vi "newfinal.vi"(8 "error in (no error)":errorcluster, 11 "output cluster in":T1) -> (0 "error out":errorcluster, 3 "output cluster out":T1)   [LabVIEW 2013]
uses:
  calib_Sub_Typdef.ctl
  ScreenCam2_TypDEf.ctl
  CamAndObj_TypDEf.ctl
  ROIInfo_TypDef.ctl
  calibPixel.ctl
  2DTypDef.ctl
  CamRoiTypDef.ctl
  finalCalibTypdef.ctl
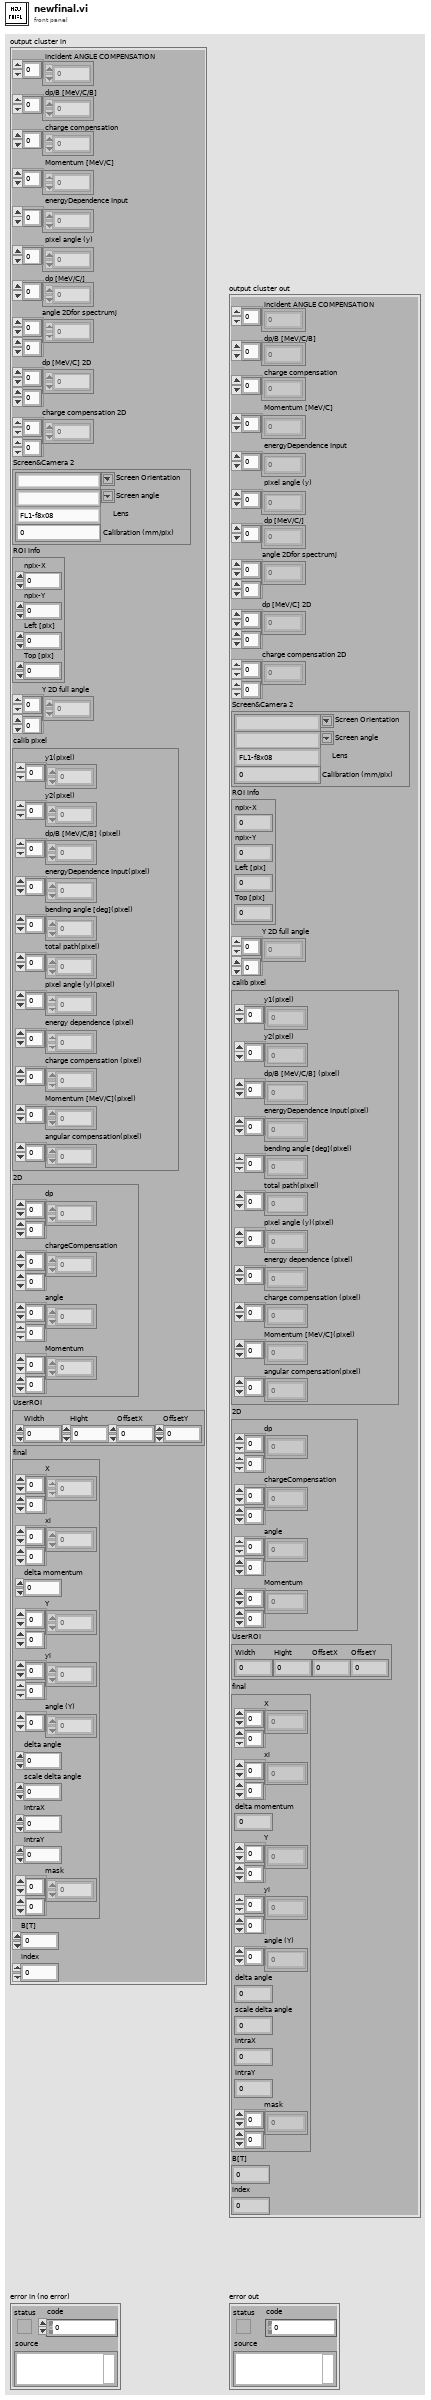
[diagram p1: front panel]
types:
  T1 = typedef "calib_Sub_Typdef.ctl" = cluster{"incident ANGLE COMPENSATION":dbl[], "dp/B [MeV/C/B]":dbl[], "charge compensation":dbl[], "Momentum [MeV/C]":dbl[], "energyDependence Input":dbl[], "pixel angle (y)":dbl[], "dp [MeV/C/] ":dbl[], "angle 2Dfor spectrumj":dbl[][], "dp [MeV/C] 2D":dbl[][], "charge compensation 2D":dbl[][], "Screen&Camera 2":T2, "ROI info":T4, "Y 2D full angle":dbl[][], "calib pixel":T5, "2D":T6, "UserROI":T7, "final":T8, "B[T]":dbl, "index":dbl}
  T2 = typedef "ScreenCam2_TypDEf.ctl" = cluster{"Screen Orientation":string, "Screen angle":string, "Lens":T3, "Calibration (mm/pix)":dbl}
  T3 = typedef "CamAndObj_TypDEf.ctl" = enum16{"FL1-f8x08", "FL1-f8x06", "FL1-f8", "ch300-f50", "FL2G-f8", "FL3M14-f8", "FL3M14-f8x08", "FL3M14-f8x08(2x2)"}
  T4 = typedef "ROIInfo_TypDef.ctl" = cluster{"npix-X":i32, "npix-Y":i32, "Left [pix]":dbl, "Top [pix]":dbl}
  T5 = typedef "calibPixel.ctl" = cluster{"y1(pixel)":dbl[], "y2(pixel)":dbl[], "dp/B [MeV/C/B] (pixel)":dbl[], "energyDependence Input(pixel)":dbl[], "bending angle [deg](pixel)":dbl[], "total path(pixel)":dbl[], "pixel angle (y)(pixel)":dbl[], "energy dependence (pixel)":dbl[], "charge compensation (pixel)":dbl[], "Momentum [MeV/C](pixel)":dbl[], "angular compensation(pixel)":dbl[]}
  T6 = typedef "2DTypDef.ctl" = cluster{"dp":dbl[][], "chargeCompensation":dbl[][], "angle":dbl[][], "Momentum":dbl[][]}
  T7 = typedef "CamRoiTypDef.ctl" = cluster{"Width":dbl, "Hight":dbl, "OffsetX":dbl, "OffsetY":dbl}
  T8 = typedef "finalCalibTypdef.ctl" = cluster{"X":dbl[][], "xi":dbl[][], "delta momentum":dbl, "Y":dbl[][], "yi":dbl[][], "angle (Y)":dbl[], "delta angle":dbl, "scale delta angle":dbl, "intraX":dbl, "intraY":dbl, "mask":dbl[][]}
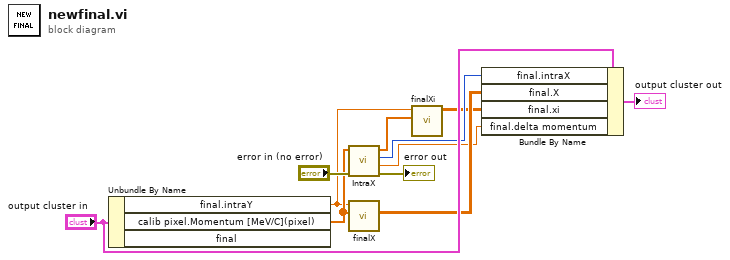
[diagram p0: block diagram]
diagram:
  n1 = Unbundle By Name("output cluster in") -> ("final.intraY"=w1:dbl, "calib pixel.Momentum [MeV/C](pixel)"=w8:dbl[])  [unwired: 1 out]
  n2 = call "IntraX.vi"("error in (no error)"="error in (no error)", "Momentum [MeV/C](pixel)"=w8) -> ("error out"=→"error out":errorcluster, "delta momentum"=w3:dbl, "IntraX"=w6:i32, "Ramp Pattern"=w9:dbl[])  [unwired: 6 in]
  n3 = call "finalX.vi"("Momentum [MeV/C](pixel)"=w8, "intraY"=w1) -> ("finalX"=w5:dbl[][])  [unwired: 9 in]
  n4 = call "finalXi.vi"("Ramp Pattern"=w9, "intraY"=w1) -> ("Array"=w4:dbl[][])  [unwired: 9 in]
  n5 = Bundle By Name(cluster="output cluster in", "final.intraX"=w6, "final.X"=w5, "final.xi"=w4, "final.delta momentum"=w3) -> (→"output cluster out":T1)
